vi "Element Events.vi"(8 "error in (no error)":errorcluster, 11 "DoubleControl in":refnum<class "SliderControl.lvclass">) -> (0 "error out":errorcluster, 2 "Element Events":refnum<class "Control Event Registrations.lvclass">, 3 "DoubleControl out":refnum<class "SliderControl.lvclass">)   [LabVIEW 2020, in "VolatusGUIElements.lvlib" / "SliderControl.lvclass"]
uses:
  SliderControl.lvclass
  C:/dev/lv20CE/relink/lv-volatus/VolatusGUI/GUI Element/GUI Element.lvclass
  C:/dev/lv20CE/relink/lv-volatus/VolatusGUI/OnValueChangeHandler/OnValueChangeHandler.lvclass
  VolatusGUI/Control Event Registrations/Control Event Registrations.lvclass
  VolatusGUI/GUI Element/GUI Element.lvclass/GUI Element.ctl
  VolatusGUI/GUI Element/GUI Element.lvclass
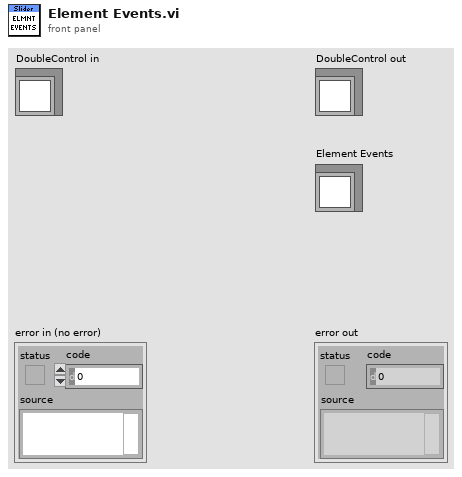
[diagram p1: front panel]
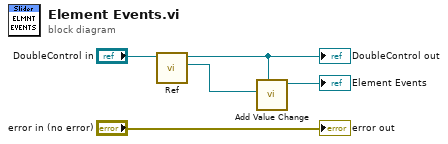
[diagram p0: block diagram]
diagram:
  n1 = call "Ref.vi"("GUI Element in"="DoubleControl in") -> ("Ref"=w1:refnum<vi>, "GUI Element out"=w2:refnum<class "SliderControl.lvclass">)  [unwired: 9 in]
  "DoubleControl out" <- w2
  n2 = call "Add Value Change.vi"("Control"=w2, "CtlRef"=w1) -> ("Control Event Registrations out"=→"Element Events":refnum<class "Control Event Registrations.lvclass">)  [unwired: 8 in, 1 out]
  "error out" <- "error in (no error)"
